vi "Write Step.vi"(8 "error in (no error)":errorcluster, 10 "Step":dbl=inf min=inf step=0.001, 11 "Voltage with Increment in":refnum<class "Voltage with Step.lvclass">) -> (0 "error out":errorcluster, 3 "Voltage with Increment out":refnum<class "Voltage with Step.lvclass">)   [LabVIEW 2023, in "HAF.lvlib" / "Voltage with Step.lvclass"]
uses:
  Voltage with Step.lvclass
  Voltage with Step.lvclass/Voltage with Step.ctl
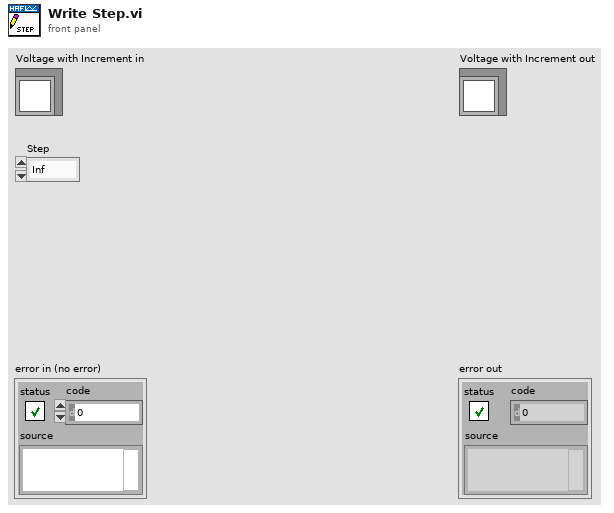
[diagram p1: front panel]
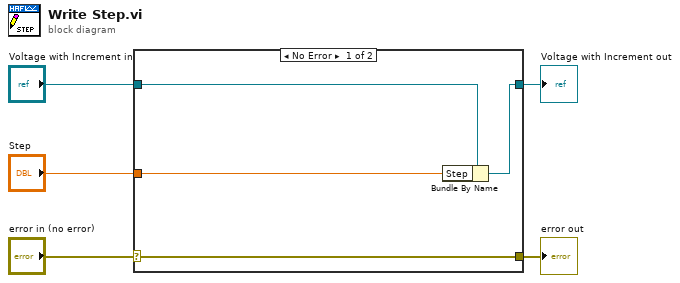
[diagram p0: block diagram]
diagram:
  n1 = case shown="No Error" "error in (no error)" {
    selector: "error in (no error)" -> [w9 w10]
    tunnel: [w9 w10] -> w4
    tunnel: [w7 w11] -> w2
    tunnel: "Voltage with Increment in" -> [w8 w11]
    tunnel: "Step" -> [w6 _]
    frame No Error {
      n2 = Bundle By Name(cluster=w8, "Step"=w6) -> (w7:refnum<class "Voltage with Step.lvclass">)
    }
    frame Error {
    }
  }
  "error out" <- w4
  "Voltage with Increment out" <- w2
